vi "Dose Correction Calculation.vi"(2 "Main Dose Calibration Cluster":T1={"Dose Response"={"grand_mean"=0.0372961188, "slope"=0.0115712882}, "Dose Correction"={"Sex"=1, "a0"=7.719669421, "a1"=-2.746550736, "a2"=-0.186490355, "a3"=0.041922063, "a4"=-0.849147359, "a5"=0.14330063, "a6"=0.019930219, "A_n"=40.0, "H_n"=10.95, "Dose Correction"=TRUE}, "Dose Reporting"={"Reporting is"=TRUE, "sd_threshold [AU]"=0.06, "sd_model [Gy]"=0.66, "dosimetric_threshold [Gy]"=2.0, "Add intrasession errors is"=TRUE, "Prior Radiation?"=TRUE}} {"Dose Reporting"."dosimetric_threshold [Gy]" format="%#_9g"; "Dose Reporting"."sd_model [Gy]" format="%#_9g"; "Dose Reporting"."sd_threshold [AU]" format="%#_9g"; "Dose Correction"."H_n" format="%#_9g"; "Dose Correction"."A_n" format="%#_9g"; "Dose Correction"."a6" format="%#.9g"; "Dose Correction"."a5" format="%#.9g"; "Dose Correction"."a4" format="%#.9g"; "Dose Correction"."a3" format="%#.9g"; "Dose Correction"."a2" format="%#.9g"; "Dose Correction"."a1" format="%#.9g"; "Dose Correction"."a0" format="%#.9g"; "Dose Correction"."Sex" items=["Male"=1, "Female"=0]; "Dose Response"."slope" format="%#_9g"; "Dose Response"."grand_mean" format="%#_9g"}, 3 "Set RIS Estimates [AU]":dbl[](array[numeric])=[0.02, 0.03, 0.04, 0.04, 0.03] format="%#_9g") -> (0 "SD_total":dbl=0.7349556237723311, 1 "RIS_Gy_corr":dbl=-0.5726655899661867)   [LabVIEW 2016]
uses:
  Dose Calculation Control.ctl
  <vilib>/Analysis/NI_AALBase.lvlib
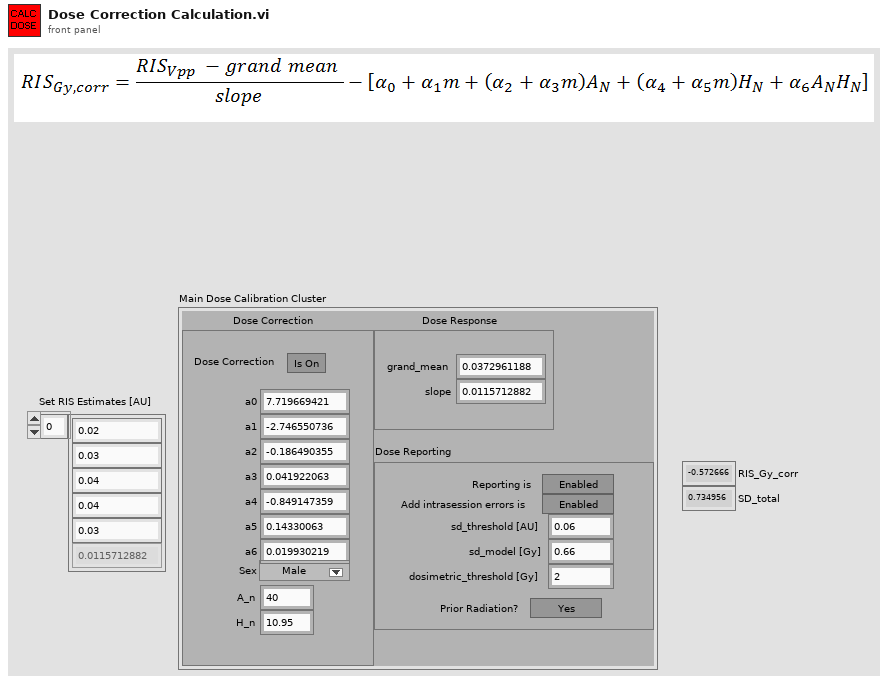
[diagram p1: front panel]
types:
  T1 = typedef "Dose Calculation Control.ctl" = cluster{"Dose Response":cluster{"grand_mean":dbl, "slope":dbl}, "Dose Correction":cluster{"Sex":u16, "a0":dbl, "a1":dbl, "a2":dbl, "a3":dbl, "a4":dbl, "a5":dbl, "a6":dbl, "A_n":dbl, "H_n":dbl, "Dose Correction":bool}, "Dose Reporting":cluster{"Reporting is":bool, "sd_threshold [AU]":dbl, "sd_model [Gy]":dbl, "dosimetric_threshold [Gy]":dbl, "Add intrasession errors is":bool, "Prior Radiation?":bool}}
  T2 = cluster{"Reporting is":bool, "sd_threshold [AU]":dbl, "sd_model [Gy]":dbl, "dosimetric_threshold [Gy]":dbl, "Add intrasession errors is":bool, "Prior Radiation?":bool}
  T3 = cluster{"Sex":u16, "a0":dbl, "a1":dbl, "a2":dbl, "a3":dbl, "a4":dbl, "a5":dbl, "a6":dbl, "A_n":dbl, "H_n":dbl, "Dose Correction":bool}
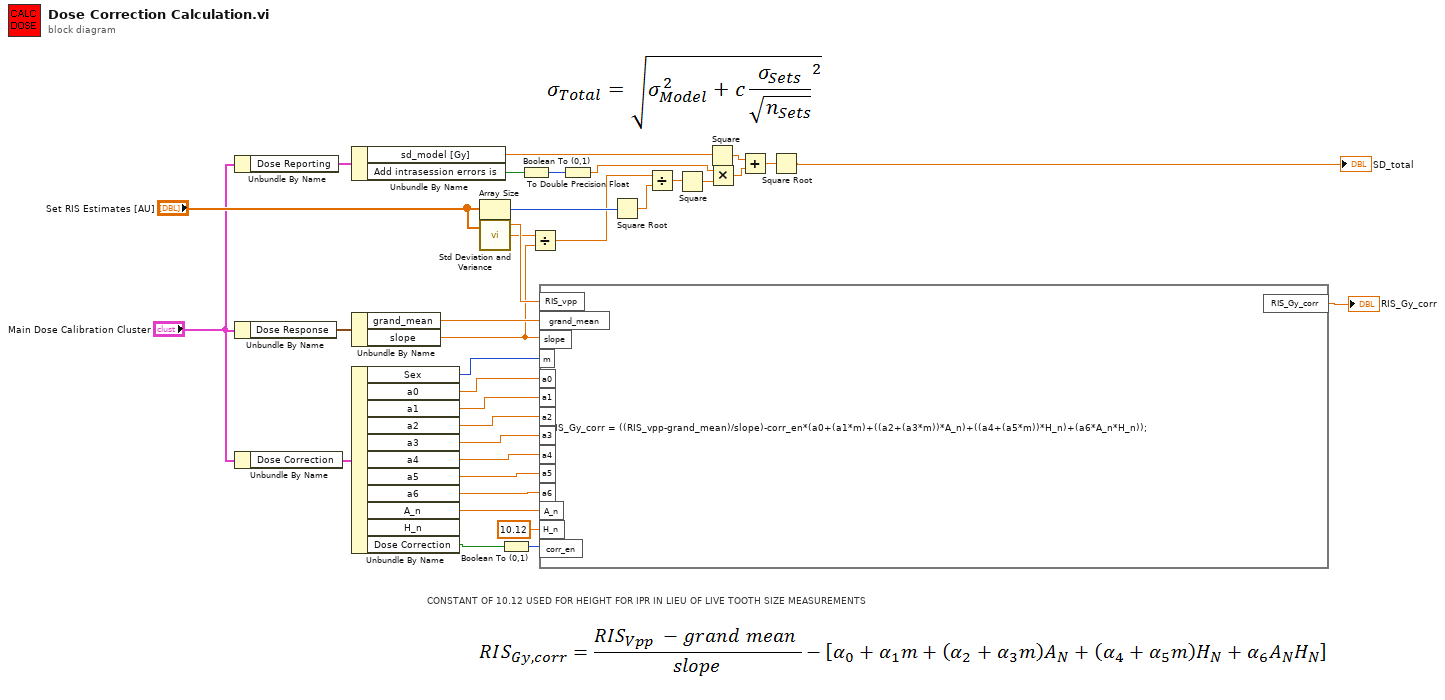
[diagram p0: block diagram]
diagram:
  # "CONSTANT OF 10.12 USED FOR HEIGHT FOR IPR IN LIEU OF LIVE TOOTH SIZE MEASUREMENTS"
  n1 = Unbundle By Name("Main Dose Calibration Cluster") -> ("Dose Reporting"=w15:T2)
  n2 = Unbundle By Name("Main Dose Calibration Cluster") -> ("Dose Response"=w17:cluster{"grand_mean":dbl, "slope":dbl})
  n3 = Unbundle By Name("Main Dose Calibration Cluster") -> ("Dose Correction"=w19:T3)
  n4 = Unbundle By Name(w15) -> ("sd_model [Gy]"=w3:dbl, "Add intrasession errors is"=w14:bool)
  n5 = Unbundle By Name(w17) -> ("grand_mean"=w18:dbl, "slope"=w13:dbl)
  n6 = Unbundle By Name(w19) -> ("Sex"=w33:u16, "a0"=w32:dbl, "a1"=w31:dbl, "a2"=w30:dbl, "a3"=w29:dbl, "a4"=w28:dbl, "a5"=w27:dbl, "a6"=w26:dbl, "A_n"=w25:dbl, "Dose Correction"=w24:bool)  [unwired: 1 out]
  n7 = Array Size(array="Set RIS Estimates [AU]") -> (size(s)=w12:i32)
  n8 = call <vilib>:"Std Deviation and Variance.vi"("X"="Set RIS Estimates [AU]") -> ("mean"=w22:dbl, "standard deviation"=w21:dbl)  [unwired: 1 in, 1 out]
  n9 = Boolean To (0,1)(Boolean=w24) -> (0, 1=w34:i16)
  n10 = Boolean To (0,1)(Boolean=w14) -> (0, 1=w7:i16)
  n11 = Divide(x=w21, y=w13) -> (x/y=w10:dbl)
  n12 = formula code="RIS_Gy_corr = ((RIS_vpp-grand_mean)/slope)-corr_en*(a0+(a1*m)+((a2+(a3*m))*A_n)+((a4+(a5*m))*H_n)+(a6*A_n*H_n));"("RIS_vpp"=w22, "grand_mean"=w18, "slope"=w13, "a0"=w32, "a1"=w31, "a2"=w30, "a3"=w29, "a4"=w28, "a5"=w27, "a6"=w26, "m"=w33, "A_n"=w25, "H_n"=10.12 ("input variable"), "corr_en"=w34) -> ("RIS_Gy_corr"=→"RIS_Gy_corr":dbl)
  n13 = To Double Precision Float(number=w7) -> (double precision float=w1:dbl)
  n14 = Square Root(x=w12) -> (sqrt(x)=w11:dbl)
  n15 = Divide(x=w10, y=w11) -> (x/y=w9:dbl)
  n16 = Square(x=w9) -> (x^2=w8:dbl)
  n17 = Square(x=w3) -> (x^2=w5:dbl)
  n18 = Multiply(x=w1, y=w8) -> (x*y=w6:dbl)
  n19 = Add(x=w5, y=w6) -> (x+y=w4:dbl)
  n20 = Square Root(x=w4) -> (sqrt(x)=→"SD_total":dbl)
